vi "TestExecuteOneShotSubscription_PublishOK.vi"(8 "error in (no error)":errorcluster, 11 "TestCase in":refnum<class "TestSubscriptionPolicy.lvclass">) -> (0 "error out":errorcluster, 3 "TestCase out":refnum<class "TestSubscriptionPolicy.lvclass">)   [LabVIEW 2015, in "TestSubscriptionPolicy.lvclass"]
uses:
  TestSubscriptionPolicy.lvclass
  Framework/SubscriptionPolicy/OneShotSubscription/OneShotSubscription.lvclass/OneShotSubscription.ctl
  Framework/SubscriptionPolicy/OneShotSubscription/OneShotSubscription.lvclass
  Framework/Transport/QueueTransport/QueueTransport.lvclass
  Framework/IMediator/ISubscriptionPolicy/ISubscriptionPolicy.lvclass
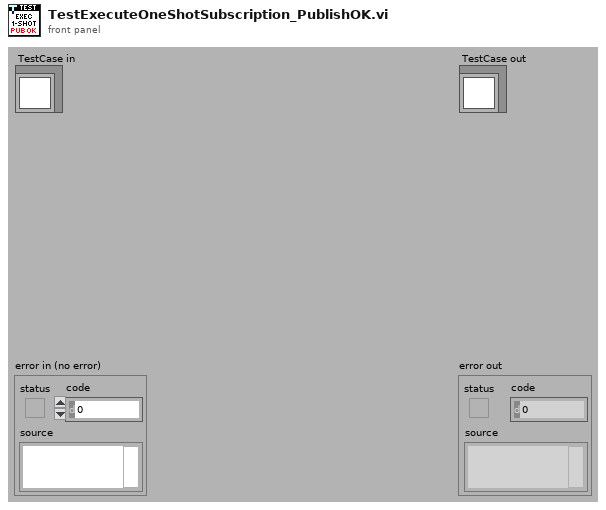
[diagram p1: front panel]
types:
  T1 = cluster{"Data":variant, "Publication Time":timestamp}
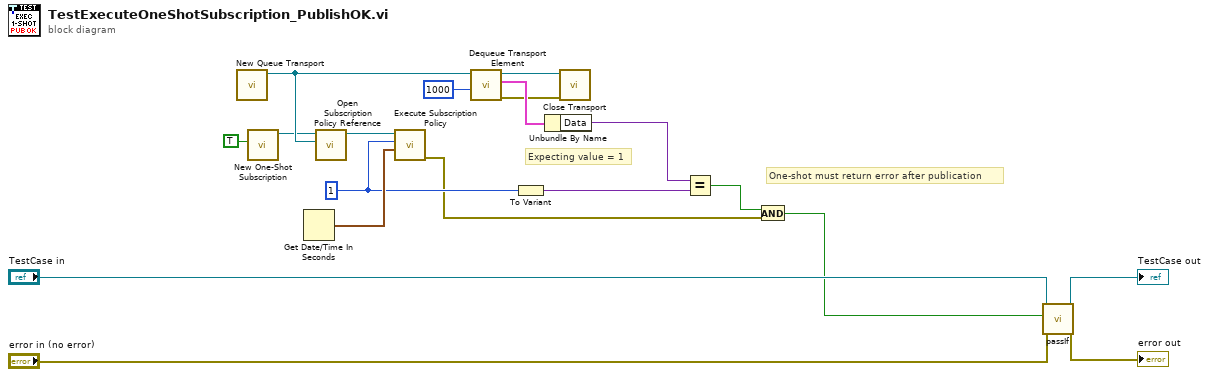
[diagram p0: block diagram]
diagram:
  w5 = 1
  # "One-shot must return error after publication"
  # "Expecting value = 1"
  n1 = call "New Queue Transport.vi"() -> ("QueueTransport Out"=w14:refnum<class "QueueTransport.lvclass">)  [unwired: 10 in, 1 out]
  n2 = call "New One-Shot Subscription.vi"("Ignore Past Updates? (F)"=TRUE) -> ("OneShotSubscription Out"=w8:refnum<class "OneShotSubscription.lvclass">)  [unwired: 10 in]
  n3 = Get Date/Time In Seconds() -> (seconds since 1Jan1904=w11:timestamp)
  n4 = call "Open Subscription Policy Reference.vi"("Transport"=w14, "SubscriptionPolicy"=w8) -> ("Subscription Policy"=w15:refnum<data-value>)  [unwired: 8 in, 1 out]
  n5 = call "Execute Subscription Policy.vi"("Publish Time"=w11, "New Topic Value"=w5, "Subscription Policy"=w15) -> ("error out (Unsubscribe?)"=w2:errorcluster)  [unwired: 8 in]
  n6 = call "Dequeue Transport Element.vi"("Timeout In ms (-1)"=1000, "QueueTransport in"=w14) -> ("error out"=w9:errorcluster, "Element"=w12:T1, "QueueTransport out"=w10:refnum<class "QueueTransport.lvclass">)  [unwired: 6 in, 1 out]
  n7 = To Variant(anything=w5) -> (Variant=w4:variant)
  n8 = Unbundle By Name(w12) -> ("Data"=w6:variant)
  n9 = call-dynamic "Close Transport.vi"("error in (no error)"=w9, "QueueTransport in"=w10) -> ()  [unwired: 9 in, 1 out]
  n10 = Equal?(x=w6, y=w4) -> (x = y?=w3:bool)
  n11 = And(x=w3, y=w2) -> (x .and. y?=w1:bool)
  n12 = call-dynamic "passIf.vi"("error in (no error)"="error in (no error)", "pass"=w1, "TestCase in"="TestCase in") -> ("error out"=→"error out":errorcluster, "TestCase out"=→"TestCase out":refnum<class "TestSubscriptionPolicy.lvclass">)  [unwired: 7 in]
